vi "Period and Phase Measurement DO.vi"() -> ()   [LabVIEW 2018]
doc: "This VI Simulates two signals at the same frequency and a user defined phase offset. These simulated inputs are then used to demonstrate the phase and measurement capability of the example. A Single Cycle Timed Loop is used."
uses:
  <vilib>/Platform/TimedLoop/XDataNode/timing_clust.ctl
  <vilib>/Platform/TimedLoop/XDataNode/nitl_modes.ctl
  <vilib>/Platform/TimedLoop/XDataNode/wakeup.ctl
  <vilib>/rvi/Emulation/niFpgaSctlEmulationGetInTimedLoop.vi
  <vilib>/rvi/Emulation/niFpgaEmulationReportErrorSimple.vi
  <vilib>/rvi/Emulation/niFpgaGetClockAttributes.vi
  <vilib>/rvi/Emulation/niFpgaCriticalErrorInLSC.vi
  <vilib>/rvi/eio/common/nirviEmuTemplateMethod_errors.vi
  <vilib>/Platform/TimedLoop/XDataNode/XDataNode.xnode
  <vilib>/eio/EIONode/EIONode.xnode
  <vilib>/Platform/TimedLoop/XDataNode/XDNodeRunTimeDep.lvlib
panel:
  out "Period (us)":u32
  out "Phase Shift (us)":u32
  out "Digital Signal B":bool
  out "Digital Signal A":bool
  # "Overview: Demonstrates Period and Phase Measurement on an FPGA\nRequirements: LabVIEW FPGA\nInstructions:\n1. Run the VI\n2. myRIO connector A/DI0(Pin 11) Signal A, A/DI1(Pin 13)  Signal B"
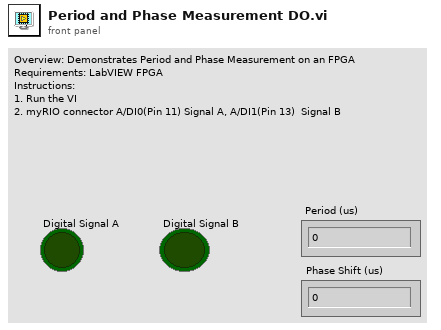
[diagram p1: front panel]
types:
  T1 = typedef "XDNodeRunTimeDep.lvlib/timing_clust.ctl" = cluster{"Expected End [f-1]":u64, "Actual End [f-1]":u64, "Finished Late? [f-1]":bool, "Expected End [i-1]":u64, "Actual End [i-1]":u64, "Finished Late? [i-1]":bool, "Expected Start [i]":u64, "Actual Start [i]":u64, "Expected Start [f]":u64, "Actual Start [f]":u64, "Source Name":string, "Structure Name":string, "Period":i64, "Deadline":i64, "Offset":i64, "Start":i64, "Priority":i32, "Timeout":i32, "Mode":T2, "Wakeup Reason":T3, "Error":errorcluster, "Source Type":string, "Secondary Source Type":string, "Global End Time":u64, "Global Start Time":u64, "Frame Duration":u64, "Iteration Duration":u64, "Assigned CPU":i32, "I/O Scan Engine Mode":u32}
  T2 = typedef "XDNodeRunTimeDep.lvlib/nitl_modes.ctl" = enum32{"No Change", "Process missed periods, maintain original phase", "Discard missed periods, maintain original phase", "Process missed periods, ignore original phase", "Discard missed periods, ignore original phase"}
  T3 = typedef "XDNodeRunTimeDep.lvlib/wakeup.ctl" = enum32{"Normal", "Aborted", "Asynchronous wakeup", "Timing source error", "Timed loop error", "Timeout"}
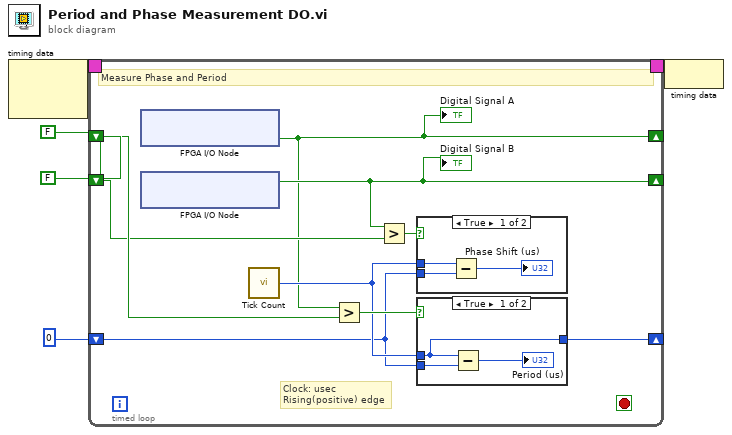
[diagram p0: block diagram]
diagram:
  n1 = node-c288() -> (w5:T1)  [unwired: 2 in]
  n2 = timed-loop "Two Edge Separation" {
    shift-left: FALSE ("Digital Signal A") -> [w13]
    shift-right: [w7] -> _
    shift-left: u32 0 ("Tick Count(Ticks)") -> [w9]
    shift-right: [w8] -> _
    shift-left: FALSE ("Digital Signal A") -> [w14]
    shift-right: [w6] -> _
    timing: w5 -> [_]
    timing-out: [_] -> w4
    stop <- _ stop-if-true
    # "Clock: usec\nRising(positive) edge"
    # "Measure Phase and Period"
    n3 = xnode "FPGA I/O Node"() -> ("ConnectorA/DIO0"=w6:bool)  [unwired: 1 in, 1 out]
    "Digital Signal A" <- w6
    n4 = xnode "FPGA I/O Node"() -> ("ConnectorA/DIO1"=w7:bool)  [unwired: 1 in, 1 out]
    "Digital Signal B" <- w7
    n5 = call "Tick Count"() -> ("Tick Count(uSec)"=w10:u32)
    n6 = Greater?(x=w6, y=w14) -> (0:w11:bool)
    n7 = Greater?(x=w7, y=w13) -> (0:w12:bool)
    n8 = case shown="True" w12 {
      tunnel: w10 -> [w20 _]
      tunnel: w9 -> [w21 _]
      frame True {
        n9 = Subtract(x=w20, y=w21) -> (x-y=→"Phase Shift (us)":u32)
      }
      frame False {
      }
    }
    n10 = case shown="True" w11 {
      tunnel: w10 -> [w15 _]
      tunnel: w9 -> [w16 w18]
      tunnel: [w15 w18] -> w8
      frame True {
        n11 = Subtract(x=w15, y=w16) -> (x-y=→"Period (us)":u32)
      }
      frame False {
      }
    }
  }
  n12 = node-c288(w4) -> ()
